vi "SwerveChooseCenter.vi"(6 "Defensive Driving Trigger":bool, 8 "Joystick Y":dbl, 9 "Joystick X":dbl) -> (3 "Center Choice":T1(ring))   [LabVIEW 2019]
doc: "***under development***"
uses:
  9a94878a-4914-4fba-839a-7657b048eec0.vi
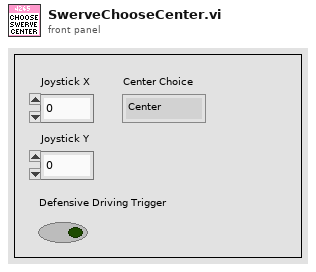
[diagram p1: front panel]
types:
  T1 = enum16{"Center", "Module 0", "Module 1", "Module 2", "Module 3"}
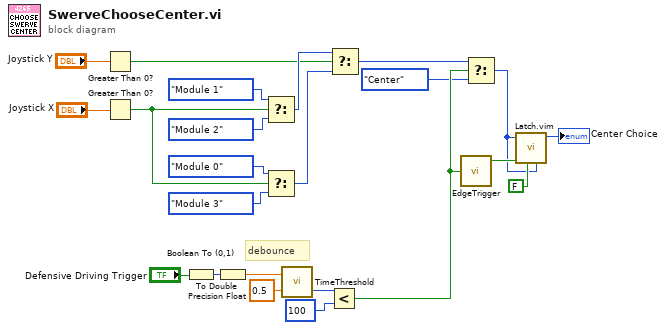
[diagram p0: block diagram]
diagram:
  # "debounce"
  n1 = Greater Than 0?(x="Joystick Y") -> (x > 0?=w20:bool)
  n2 = Greater Than 0?(x="Joystick X") -> (x > 0?=w22:bool)
  n3 = Boolean To (0,1)(Boolean="Defensive Driving Trigger") -> (0, 1=w13:i16)
  n4 = To Double Precision Float(number=w13) -> (double precision float=w12:dbl)
  n5 = Select(t=T1."Module 1", s=w22, f=T1."Module 2") -> (s? t:f=w21:T1)
  n6 = Select(t=T1."Module 0", s=w22, f=T1."Module 3") -> (s? t:f=w23:T1)
  n7 = call "TimeThreshold.vi"("Threshold"=0.5, "Current Value"=w12) -> ("Time Below Threshold (ms)"=w11:u32)  [unwired: 1 out]
  n8 = Less?(x=w11, y=u32 100) -> (x < y?=w9:bool)
  n9 = Select(t=w21, s=w20, f=w23) -> (s? t:f=w5:T1)
  n10 = call "EdgeTrigger.vi"("Input Signal"=w9) -> ("Rising Edge Trigger"=w17:bool)  [unwired: 2 out]
  n11 = Select(t=w5, s=w9, f=T1."Center") -> (s? t:f=w7:T1)
  n12 = call "Latch.vim"("Default Value"=w7, "Reset"=FALSE, "Latch Signal"=w17, "Latch Value"=w7) -> ("Latched"=→"Center Choice":T1)  [unwired: 7 in]
